vi "Create.vi"(7 "Alpha":dbl, 8 "error in (no error)":errorcluster, 9 "Image Size":T1, 11 "Camera Parameters in":T3) -> (0 "error out":errorcluster, 1 "Valid Pixels Size":T1, 2 "New Camera Parameters":T3, 3 "New ImageRectifier":refnum<class "ImageRectifier.lvclass">, 5 "Valid Pixels Top Left":T2)   [LabVIEW 2020, in "image.lvlib" / "ImageRectifier.lvclass"]
uses:
  ImageRectifier.lvclass
  common/Camera Parameters.ctl
  common/Camera Matrix.ctl
  common/Camera Distortion Coefficients.ctl
  common/Image Size (Integer).ctl
  common/Image Point (Integer).ctl
  ImageRectifier.lvclass/ImageRectifier.ctl
  common/common.lvlib
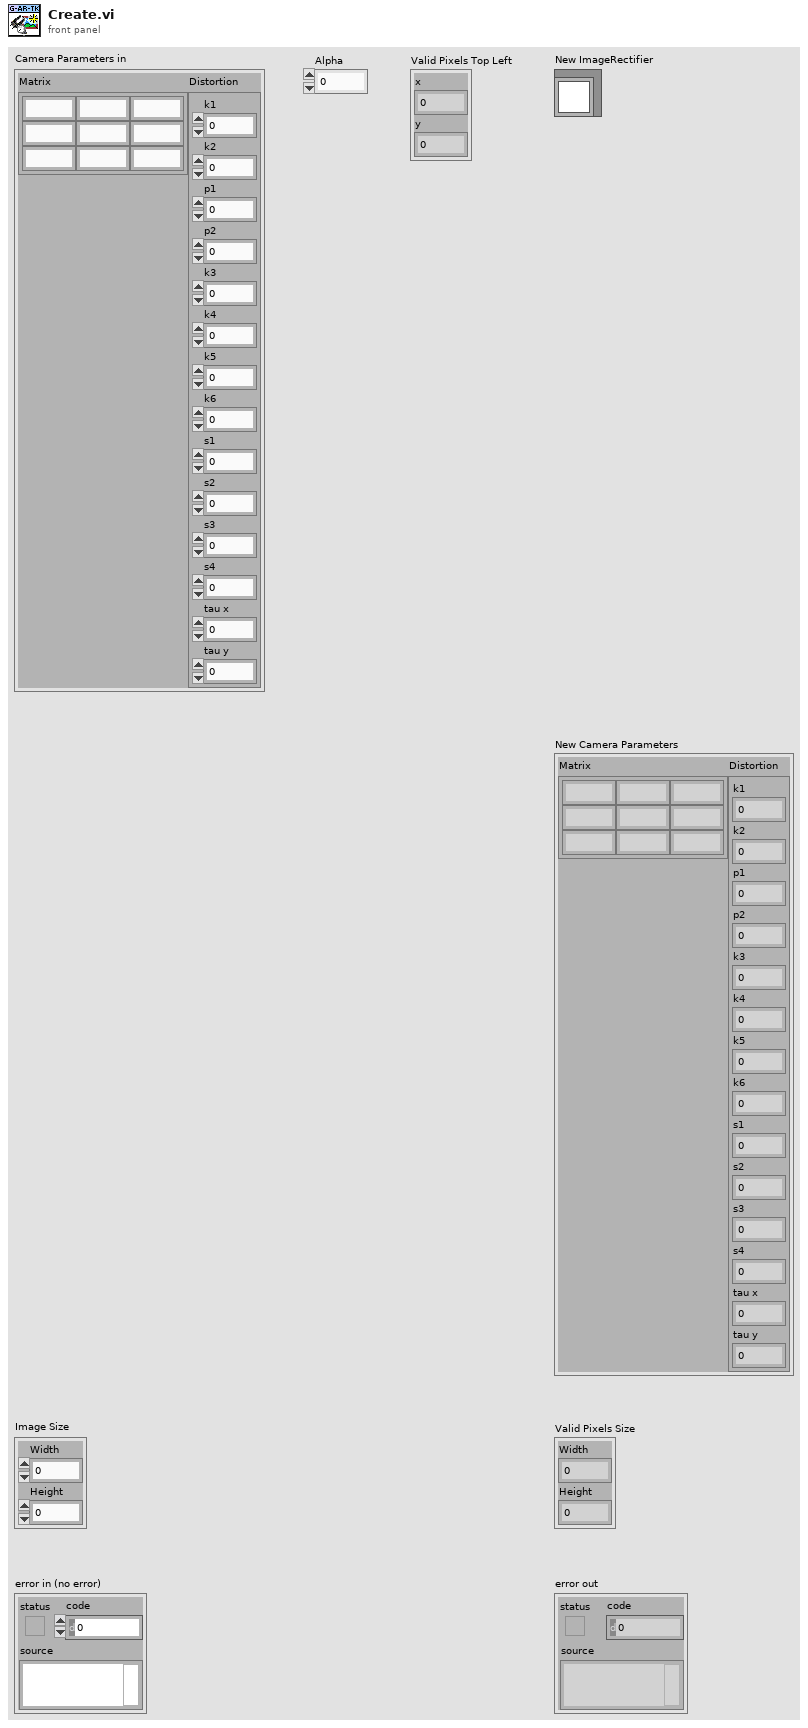
[diagram p1: front panel]
types:
  T1 = typedef "common.lvlib/Image Size (Integer).ctl" = cluster{"Width":u16, "Height":u16}
  T2 = typedef "common.lvlib/Image Point (Integer).ctl" = cluster{"x":i32, "y":i32}
  T3 = typedef "common.lvlib/Camera Parameters.ctl" = cluster{"Matrix":T4, "Distortion":T5}
  T4 = typedef "common.lvlib/Camera Matrix.ctl" = cluster{"m 0,0":dbl, "m 0,1":dbl, "m 0,2":dbl, "m 1,0":dbl, "m 1,1":dbl, "m 1,2":dbl, "m 2,0":dbl, "m 2,1":dbl, "m 2,2":dbl}
  T5 = typedef "common.lvlib/Camera Distortion Coefficients.ctl" = cluster{"k1":dbl, "k2":dbl, "p1":dbl, "p2":dbl, "k3":dbl, "k4":dbl, "k5":dbl, "k6":dbl, "s1":dbl, "s2":dbl, "s3":dbl, "s4":dbl, "tau x":dbl, "tau y":dbl}
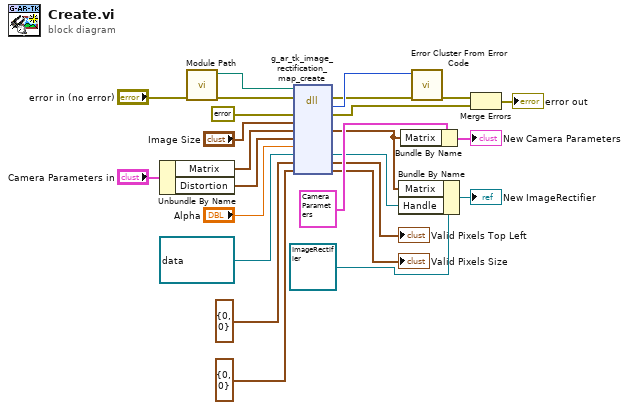
[diagram p0: block diagram]
diagram:
  n1 = Unbundle By Name("Camera Parameters in") -> ("Matrix"=w15:T4, "Distortion"=w14:T5)
  n2 = call "Module Path.vi"("error in (no error)"="error in (no error)") -> ("error out"=w20:errorcluster, "Path"=w19:path)  [unwired: 9 in]
  n3 = dll-call lib="?" fn="g_ar_tk_image_rectification_map_create" ("g_ar_toolkit.*.*:g_ar_tk_image_add_weighted")(path in=w19, error in=w20, "error_cluster"=errorcluster {"status"=FALSE, "code"=0, "source"=""} ("error constant"), "size"="Image Size", "camera_matrix"=w15, "distortion_param"=w14, "alpha"="Alpha", "EDVR"=refnum<data-value> refnum, "roi_top_left"=T2 {"x"=0, "y"=0} ("Image Point"), "roi_size"=T1 {"Width"=0, "Height"=0} ("roi_bottom_right")) -> (error out=w21:errorcluster, "MgErr"=w22:i32, "error_cluster"=w25:errorcluster, "camera_matrix"=w1:T4, "EDVR"=w9:refnum<data-value>, "roi_top_left"=→"Valid Pixels Top Left":T2, "roi_size"=→"Valid Pixels Size":T1)  [unwired: 4 in, 1 out]
  n4 = Bundle By Name(cluster=refnum<class "ImageRectifier.lvclass"> refnum ("ImageRectifier out"), "Matrix"=w1, "Handle"=w9) -> (→"New ImageRectifier":refnum<class "ImageRectifier.lvclass">)
  n5 = Bundle By Name(cluster=T3 {"Matrix"={"m 0,0"=0.0, "m 0,1"=0.0, "m 0,2"=0.0, "m 1,0"=0.0, "m 1,1"=0.0, "m 1,2"=0.0, "m 2,0"=0.0, "m 2,1"=0.0, "m 2,2"=0.0}, "Distortion"={"k1"=0.0, "k2"=0.0, "p1"=0.0, "p2"=0.0, "k3"=0.0, "k4"=0.0, "k5"=0.0, "k6"=0.0, "s1"=0.0, "s2"=0.0, "s3"=0.0, "s4"=0.0, "tau x"=0.0, "tau y"=0.0}} ("Camera Parameters in"), "Matrix"=w1) -> (→"New Camera Parameters":T3)
  n6 = call <vilib>:"Error Cluster From Error Code.vi"("error in (no error)"=w21, "error code (0)"=w22) -> ("error out"=w23:errorcluster)  [unwired: 7 in]
  n7 = Merge Errors(w23, w25) -> (→"error out":errorcluster)
